vi "Test Skip Overrides Upstreams Error Status.vi"(8 "error in (no error)":errorcluster, 11 "Test Assertion Results in":refnum<class "Assertion Result Test.lvclass">) -> (0 "error out":errorcluster, 3 "Test Assertion Results out":refnum<class "Assertion Result Test.lvclass">)   [LabVIEW 2020, in "LUnit Tests.lvlib" / "Assertion Result Test.lvclass"]
uses:
  Assertion Result Test.lvclass
  Test Dummys/Test Case Test Double/Test Case Test Double.lvclass
  source/Framework/Test Case/LUnit Test Case.lvclass
  source/Framework/Result Types/Case Result/Test Case Result.lvlib
  <vilib>/Astemes/LUnit/Test Case.lvclass
  source/Framework/Result Types/Assertion Result/Public/TypeDefs/Status.ctl
  source/Framework/Result Types/Assertion Result/Assertion Result.lvlib
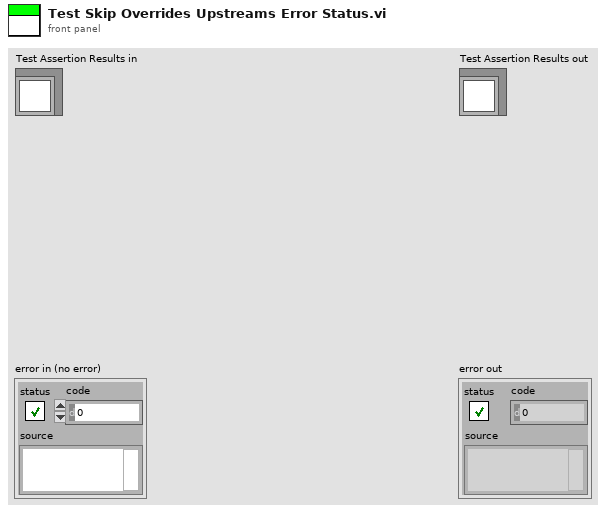
[diagram p1: front panel]
types:
  T1 = typedef "Assertion Result.lvlib/Status.ctl" = enum16{"Pass", "Fail", "Error", "Skipped", "Setup Error", "Broken", "Teardown Error"}
  T2 = typedef "Test Case Result.lvlib/Test Case Result.ctl" = map{string, T3}
  T3 = typedef "Method Result.lvlib/Method Result.ctl" = cluster{"Test Case":string, "Test Method Name":string, "Status":T1, "Assertion Results":T4[], "Execution time":dbl, "Result String":string}
  T4 = typedef "Assertion Result.lvlib/Assertion Result.ctl" = cluster{"Status":T1, "Message":string, "Description":string, "Assertion Type":T5}
  T5 = typedef "Assertion Result.lvlib/Assertion Type.ctl" = enum16{"None", "Pass", "Fail", "Skip", "Pass if Equal", "Fail if Equal", "Pass if Error", "Fail if Error", "Pass if", "Fail if"}
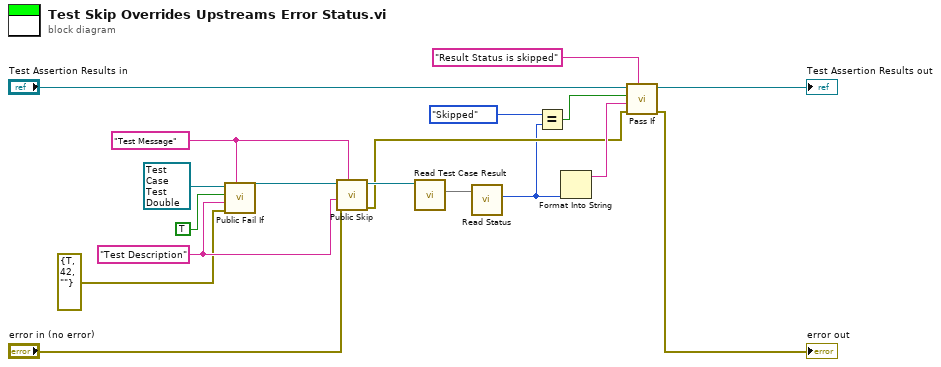
[diagram p0: block diagram]
diagram:
  w13 = "Test Message" ("Description")
  w14 = "Test Description" ("Description")
  n1 = call "Public Fail If.vi"("Message"=w13, "error in (no error)"=errorcluster {"status"=TRUE, "code"=42, "source"=""}, "Description"=w14, "Fail?"=TRUE, "Test Case Test Double in"=refnum<class "Test Case Test Double.lvclass"> refnum ("Test Case Test Double.lvclass")) -> ("Test Case Test Double out"=w15:refnum<class "Test Case Test Double.lvclass">)  [unwired: 5 in, 1 out]
  n2 = call "Public Skip.vi"("Description"=w13, "error in (no error)"="error in (no error)", "Message"=w14, "Test Case Test Double in"=w15) -> ("error out"=w7:errorcluster, "Test Case Test Double out"=w12:refnum<class "Test Case Test Double.lvclass">)  [unwired: 6 in]
  n3 = call "Read Test Case Result.vi"("LUnit Test Case In"=w12) -> ("Test Case Result"=w11:T2)  [unwired: 9 in, 1 out]
  n4 = call "Read Status.vi"("Test Case Result In"=w11) -> ("Status"=w5:T1)  [unwired: 8 in, 2 out]
  n5 = Equal?(x=Status."Skipped" ("y"), y=w5) -> (x = y?=w3:bool)
  n6 = Format Into String(w5) -> (resulting string=w8:string)  [unwired: 3 in, 1 out]
  n7 = call <vilib>:"Pass If.vi"("Description"="Result Status is skipped", "error in (no error)"=w7, "Message"=w8, "Pass?"=w3, "LUnit Test Case In"="Test Assertion Results in") -> ("error out"=→"error out":errorcluster, "LUnit Test Case Out"=→"Test Assertion Results out":refnum<class "Assertion Result Test.lvclass">)  [unwired: 5 in]
